vi "Motion Path Planing Sub_VI.vi"(2 "Motion Planning Inputs":T2) -> (5 "No-limit Velocity":dbl, 6 "Motion Profile":T3=enum."Triangular", 7 "Motion Planning Outputs":T1)   [LabVIEW 2017]
uses:
  Motion Type Def.ctl
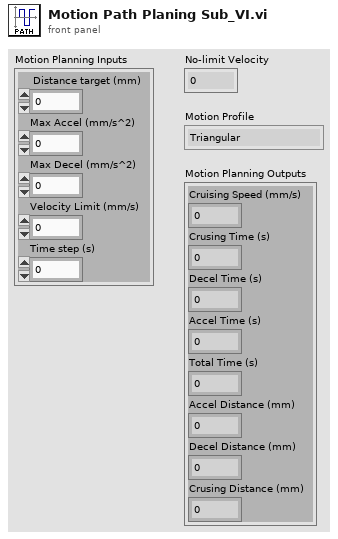
[diagram p1: front panel]
types:
  T1 = cluster{"Cruising Speed (mm/s)":dbl, "Crusing Time (s)":dbl, "Decel Time (s)":dbl, "Accel Time (s)":dbl, "Total Time (s)":dbl, "Accel Distance (mm)":dbl, "Decel Distance (mm)":dbl, "Crusing Distance (mm)":dbl}
  T2 = cluster{" Distance target (mm)":dbl, "Max Accel (mm/s^2)":dbl, "Max Decel (mm/s^2)":dbl, "Velocity Limit (mm/s) ":dbl, "Time step (s)":dbl}
  T3 = typedef "Motion Type Def.ctl" = enum16{"Trapezodial", "Triangular"}
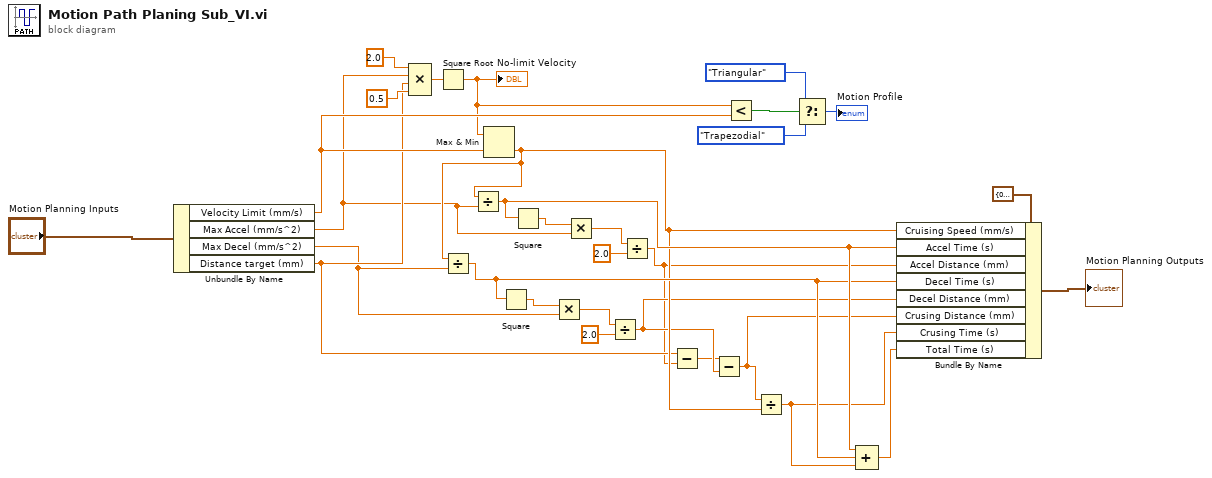
[diagram p0: block diagram]
diagram:
  n1 = Unbundle By Name("Motion Planning Inputs") -> ("Velocity Limit (mm/s)"=w23:dbl, "Max Accel (mm/s^2)"=w14:dbl, "Max Decel (mm/s^2)"=w7:dbl, "Distance target (mm)"=w15:dbl)
  n2 = Compound Arithmetic op=MULTIPLY(2.0 ("value"), w14, w15, 0.5 ("value")) -> (w17:dbl)
  n3 = Square Root(x=w17) -> (sqrt(x)=w22:dbl)
  "No-limit Velocity" <- w22
  n4 = Max & Min(x=w22, y=w23) -> (min(x,y)=w18:dbl)  [unwired: 1 out]
  n5 = Divide(x=w18, y=w7) -> (x/y=w19:dbl)
  n6 = Divide(x=w18, y=w14) -> (x/y=w20:dbl)
  n7 = Square(x=w19) -> (x^2=w4:dbl)
  n8 = Square(x=w20) -> (x^2=w3:dbl)
  n9 = Multiply(x=w4, y=w7) -> (x*y=w5:dbl)
  n10 = Multiply(x=w3, y=w14) -> (x*y=w2:dbl)
  n11 = Divide(x=w5, y=2.0) -> (x/y=w10:dbl)
  n12 = Divide(x=w2, y=2.0) -> (x/y=w9:dbl)
  n13 = Subtract(x=w15, y=w9) -> (x-y=w8:dbl)
  n14 = Subtract(x=w8, y=w10) -> (x-y=w11:dbl)
  n15 = Less?(x=w22, y=w23) -> (x < y?=w24:bool)
  n16 = Divide(x=w11, y=w18) -> (x/y=w12:dbl)
  n17 = Select(t=Motion_Type_Def."Triangular", s=w24, f=Motion_Type_Def."Trapezodial") -> (s? t:f=→"Motion Profile":T3)
  n18 = Compound Arithmetic op=ADD(w20, w19, w12) -> (w21:dbl)
  n19 = Bundle By Name(cluster=T1 {"Cruising Speed (mm/s)"=0.0, "Crusing Time (s)"=0.0, "Decel Time (s)"=0.0, "Accel Time (s)"=0.0, "Total Time (s)"=0.0, "Accel Distance (mm)"=0.0, "Decel Distance (mm)"=0.0, "Crusing Distance (mm)"=0.0} ("Motion Planning Outputs 2"), "Cruising Speed (mm/s)"=w18, "Accel Time (s)"=w20, "Accel Distance (mm)"=w9, "Decel Time (s)"=w19, "Decel Distance (mm)"=w10, "Crusing Distance (mm)"=w11, "Crusing Time (s)"=w12, "Total Time (s)"=w21) -> (→"Motion Planning Outputs":T1)
